vi "vendingmachine.vi"() -> ()   [LabVIEW 2024]
panel:
  out "s? t:f":string
  out "Coke light":bool
  out "Water light":bool
  out "Chocolate light":bool
  out "chips light":bool
  out "2 zl light":bool
  in  "2 zl":bool
  in  "Chips":bool
  in  "Chocolate":bool
  in  "Water":bool
  out "1 light":bool
  out "50 light":bool
  out "25 light":bool
  in  "Cancel Button":bool
  out "Change":string
  out "Balance":string
  in  "0.25 zl":bool
  in  "Coke":bool
  in  "1 zl":bool
  in  "0.5 zl":bool
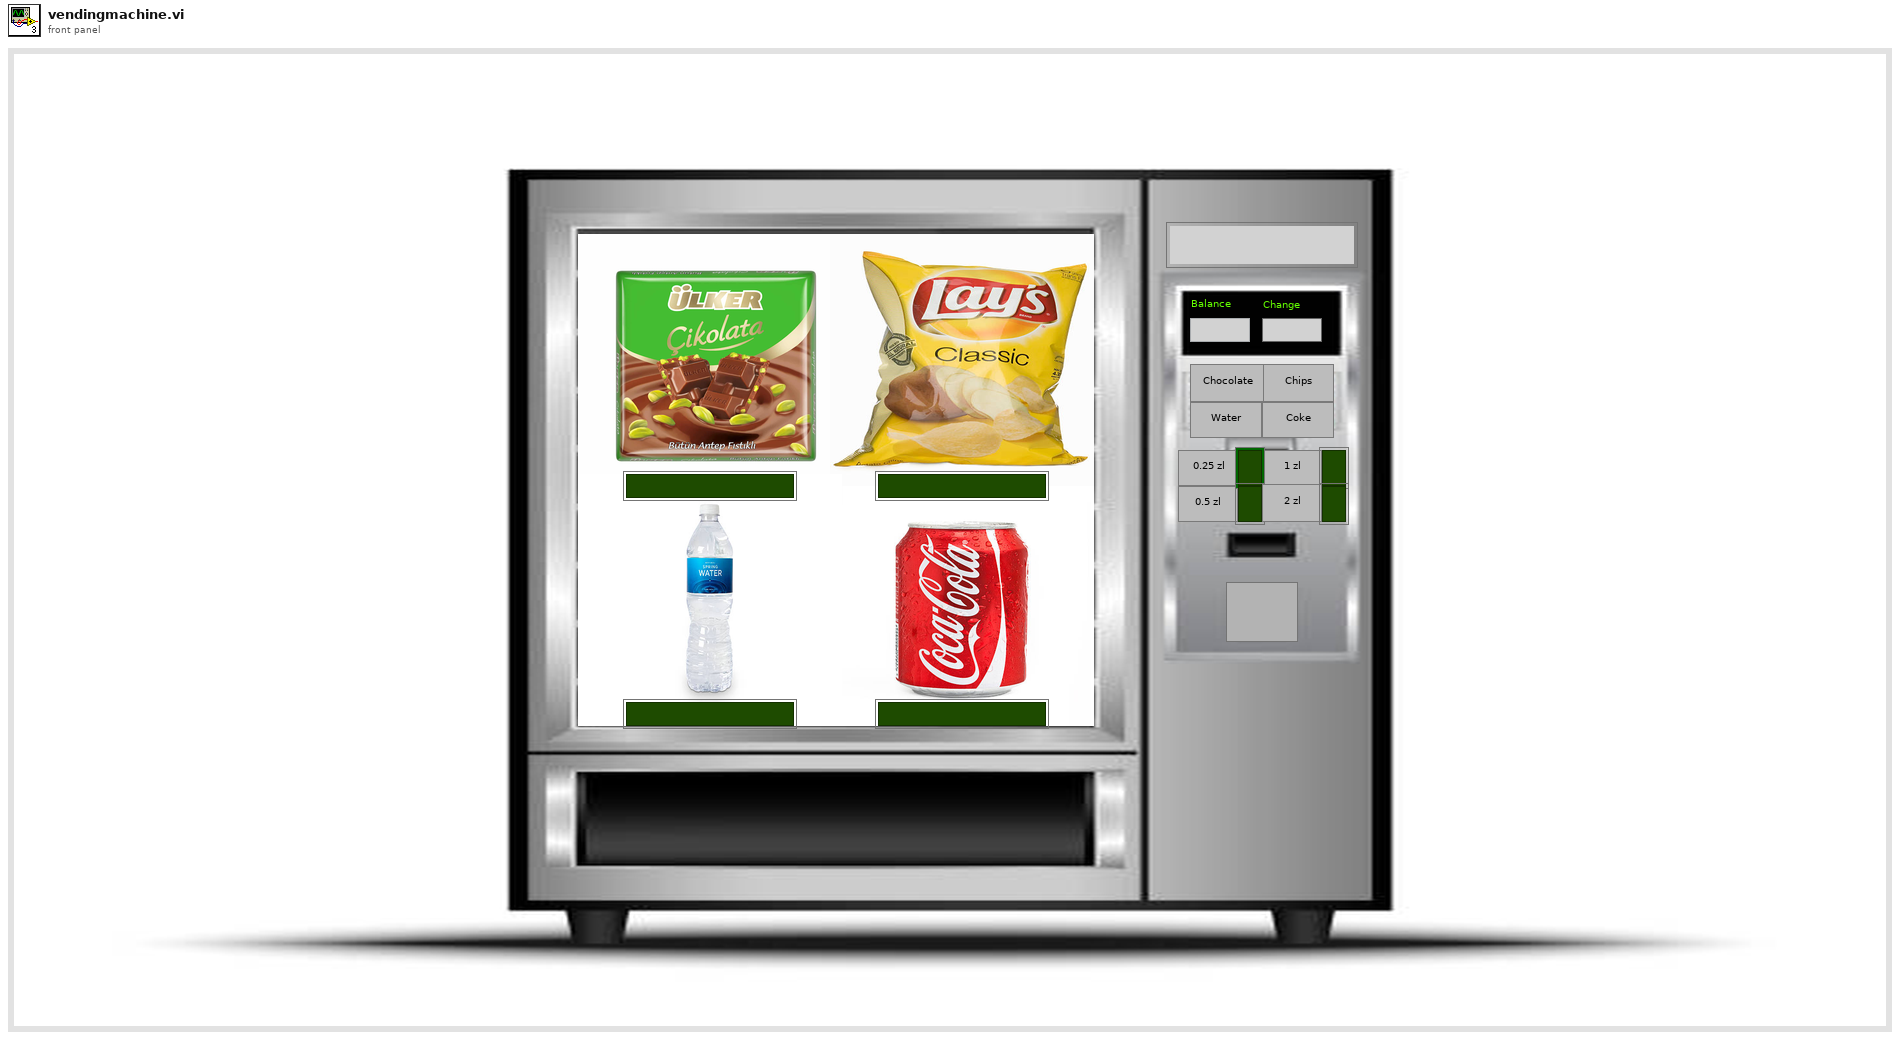
[diagram p1: front panel]
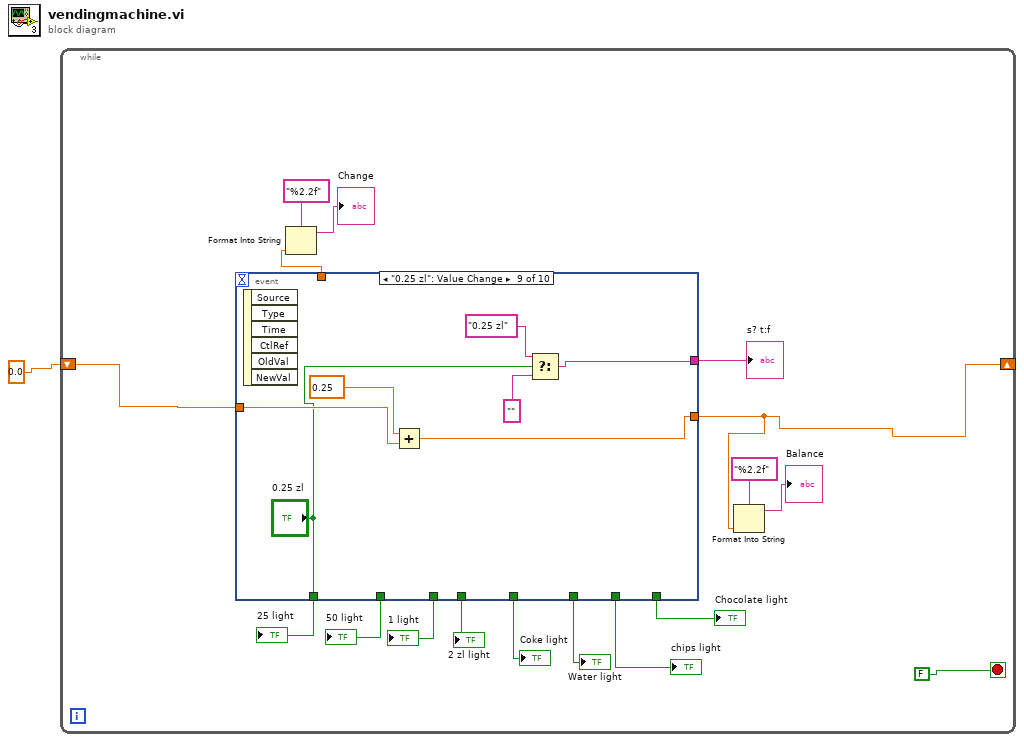
[diagram p0: block diagram]
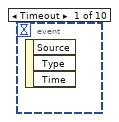
[diagram p2: hidden frame]
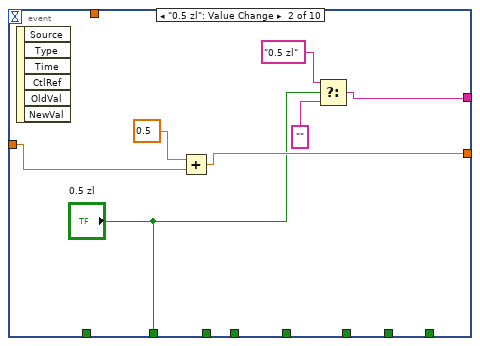
[diagram p3: hidden frame]
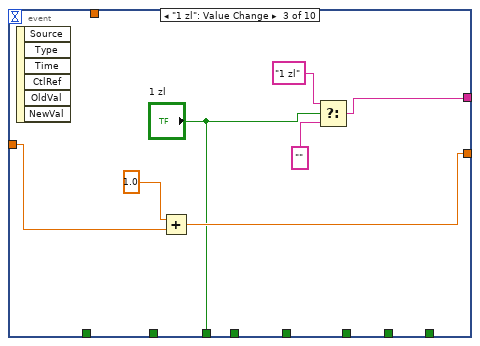
[diagram p4: hidden frame]
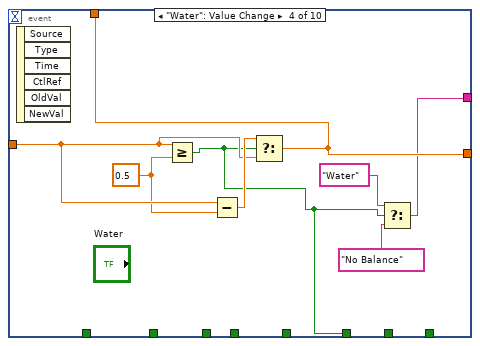
[diagram p5: hidden frame]
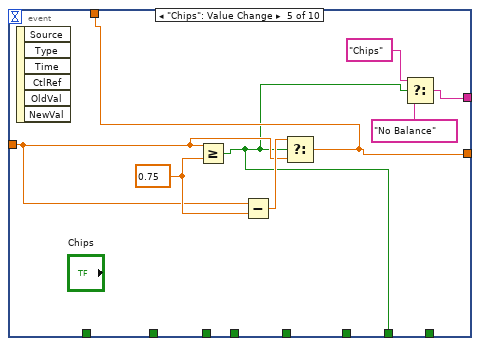
[diagram p6: hidden frame]
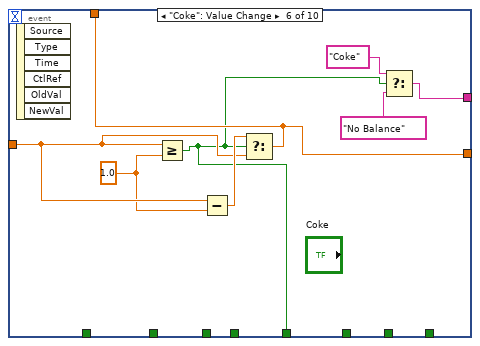
[diagram p7: hidden frame]
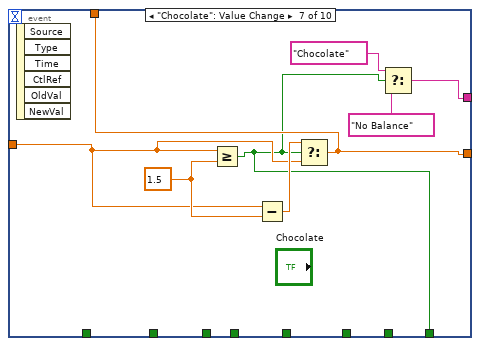
[diagram p8: hidden frame]
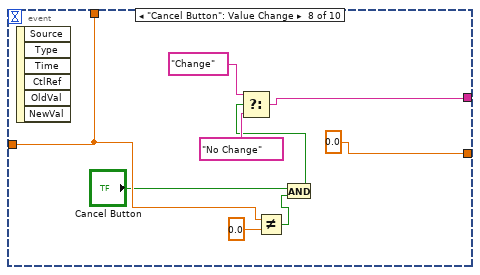
[diagram p9: hidden frame]
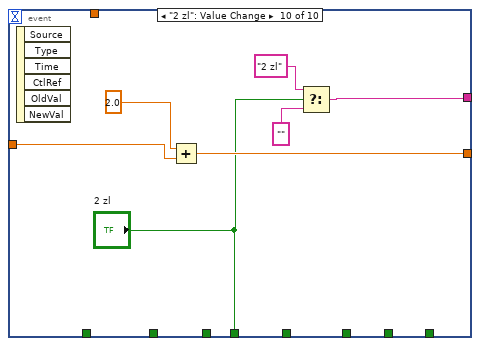
[diagram p10: hidden frame]
diagram:
  n1 = while {
    shift-right: [w15] -> _
    shift-left: 0.0 -> [w16]
    stop <- FALSE stop-if-true
    n2 = event shown="[8] \"0.25 zl\": Value Change" {
      selector: _ -> [_ _ _ _ _ _ _ _ _ _]
      dyn-events: _ -> [_ _ _ _ _ _ _ _ _ _]
      timeout: _ -> [_ _ _ _ _ _ _ _ _ _]
      tunnel: w16 -> [_ w25 w31 w39 w46 w55 w62 w69 w80 w85]
      tunnel: [_ w23 w30 w38 w45 w54 w61 0.0 w78 w86] -> w15
      tunnel: [_ _ _ w38 w45 w54 w61 w69 _ _] -> w12
      tunnel: [_ _ _ _ _ _ _ _ "0.25 zl" _] -> w11
      tunnel: [_ "0.5 zl" _ _ _ _ _ _ _ _] -> w10
      tunnel: [_ _ "1 zl" _ _ _ _ _ _ _] -> w9
      tunnel: [_ _ _ _ _ _ _ _ _ "2 zl"] -> w7
      tunnel: [_ _ _ w36 _ _ _ _ _ _] -> w6
      tunnel: [_ _ _ _ w41 _ _ _ _ _] -> w5
      tunnel: [_ _ _ _ _ w49 _ _ _ _] -> w4
      tunnel: [_ _ _ _ _ _ w57 _ _ _] -> w3
      tunnel: [_ w20 w26 w33 w42 w50 w58 w70 w75 w82] -> w2
      event Timeout {
        n3 = event-data() -> ()  [unwired: 1 in, 3 out]
      }
      event "0.5 zl": Value Change {
        n4 = event-data() -> ()  [unwired: 1 in, 6 out]
        n5 = Add(x=0.5 ("f"), y=w25) -> (x+y=w23:dbl)
        n6 = Select(t="0.5 zl" ("String"), s="0.5 zl", f="" ("String")) -> (s? t:f=w20:string)
      }
      event "1 zl": Value Change {
        n7 = event-data() -> ()  [unwired: 1 in, 6 out]
        n8 = Add(x=1.0 ("f"), y=w31) -> (x+y=w30:dbl)
        n9 = Select(t="1 zl" ("String"), s="1 zl", f="" ("String")) -> (s? t:f=w26:string)
      }
      event "Water": Value Change {
        w37 = 0.5 ("y")
        n10 = event-data() -> ()  [unwired: 1 in, 6 out]
        n11 = Greater Or Equal?(x=w39, y=w37) -> (x >= y?=w36:bool)
        n12 = Subtract(x=w39, y=w37) -> (x-y=w40:dbl)
        n13 = Select(t=w40, s=w36, f=w39) -> (s? t:f=w38:dbl)
        n14 = Select(t="Water" ("String"), s=w36, f="No Balance" ("String")) -> (s? t:f=w33:string)
      }
      event "Chips": Value Change {
        w47 = 0.75 ("y")
        n15 = event-data() -> ()  [unwired: 1 in, 6 out]
        n16 = Greater Or Equal?(x=w46, y=w47) -> (x >= y?=w41:bool)
        n17 = Subtract(x=w46, y=w47) -> (x-y=w48:dbl)
        n18 = Select(t=w48, s=w41, f=w46) -> (s? t:f=w45:dbl)
        n19 = Select(t="Chips" ("String"), s=w41, f="No Balance" ("String")) -> (s? t:f=w42:string)
      }
      event "Coke": Value Change {
        w53 = 1.0 ("y")
        n20 = event-data() -> ()  [unwired: 1 in, 6 out]
        n21 = Greater Or Equal?(x=w55, y=w53) -> (x >= y?=w49:bool)
        n22 = Subtract(x=w55, y=w53) -> (x-y=w56:dbl)
        n23 = Select(t=w56, s=w49, f=w55) -> (s? t:f=w54:dbl)
        n24 = Select(t="Coke" ("String"), s=w49, f="No Balance" ("String")) -> (s? t:f=w50:string)
      }
      event "Chocolate": Value Change {
        w63 = 1.5 ("y")
        n25 = event-data() -> ()  [unwired: 1 in, 6 out]
        n26 = Greater Or Equal?(x=w62, y=w63) -> (x >= y?=w57:bool)
        n27 = Subtract(x=w62, y=w63) -> (x-y=w64:dbl)
        n28 = Select(t=w64, s=w57, f=w62) -> (s? t:f=w61:dbl)
        n29 = Select(t="Chocolate" ("String"), s=w57, f="No Balance" ("String")) -> (s? t:f=w58:string)
      }
      event "Cancel Button": Value Change {
        n30 = event-data() -> ()  [unwired: 1 in, 6 out]
        n31 = Not Equal?(x=w69, y=0.0) -> (x != y?=w66:bool)
        n32 = And(x="Cancel Button", y=w66) -> (x .and. y?=w65:bool)
        n33 = Select(t="Change" ("String"), s=w65, f="No Change" ("String")) -> (s? t:f=w70:string)
      }
      event "0.25 zl": Value Change {
        n34 = event-data() -> ()  [unwired: 1 in, 6 out]
        n35 = Add(x=0.25 ("f"), y=w80) -> (x+y=w78:dbl)
        n36 = Select(t="0.25 zl" ("String"), s="0.25 zl", f="" ("String")) -> (s? t:f=w75:string)
      }
      event "2 zl": Value Change {
        n37 = event-data() -> ()  [unwired: 1 in, 6 out]
        n38 = Add(x=2.0 ("f"), y=w85) -> (x+y=w86:dbl)
        n39 = Select(t="2 zl" ("String"), s="2 zl", f="" ("String")) -> (s? t:f=w82:string)
      }
    }
    "25 light" <- w11
    "1 light" <- w9
    "50 light" <- w10
    "Coke light" <- w4
    "Water light" <- w6
    "Chocolate light" <- w3
    "chips light" <- w5
    "2 zl light" <- w7
    "s? t:f" <- w2
    n40 = Format Into String(format string="%2.2f", w12) -> (resulting string=→"Change":string)  [unwired: 2 in, 1 out]
    n41 = Format Into String(format string="%2.2f", w15) -> (resulting string=→"Balance":string)  [unwired: 2 in, 1 out]
  }
